vi "Main.vi"() -> ()   [LabVIEW 2015]
uses:
  Share Data/DEVICE_BUSY.ctl
  Share Data/Share Variable.lvlib
panel:
  out "elements":string[](array[string])
  out "Command":string
  out "String 2":string
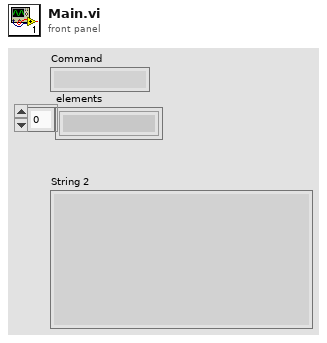
[diagram p1: front panel]
types:
  T1 = typedef "DEVICE_BUSY.ctl" = cluster{"DEV":string, "BUSY":bool, "VBAT":dbl, "OUTPUT":bool, "LAST_RESULT":dbl}
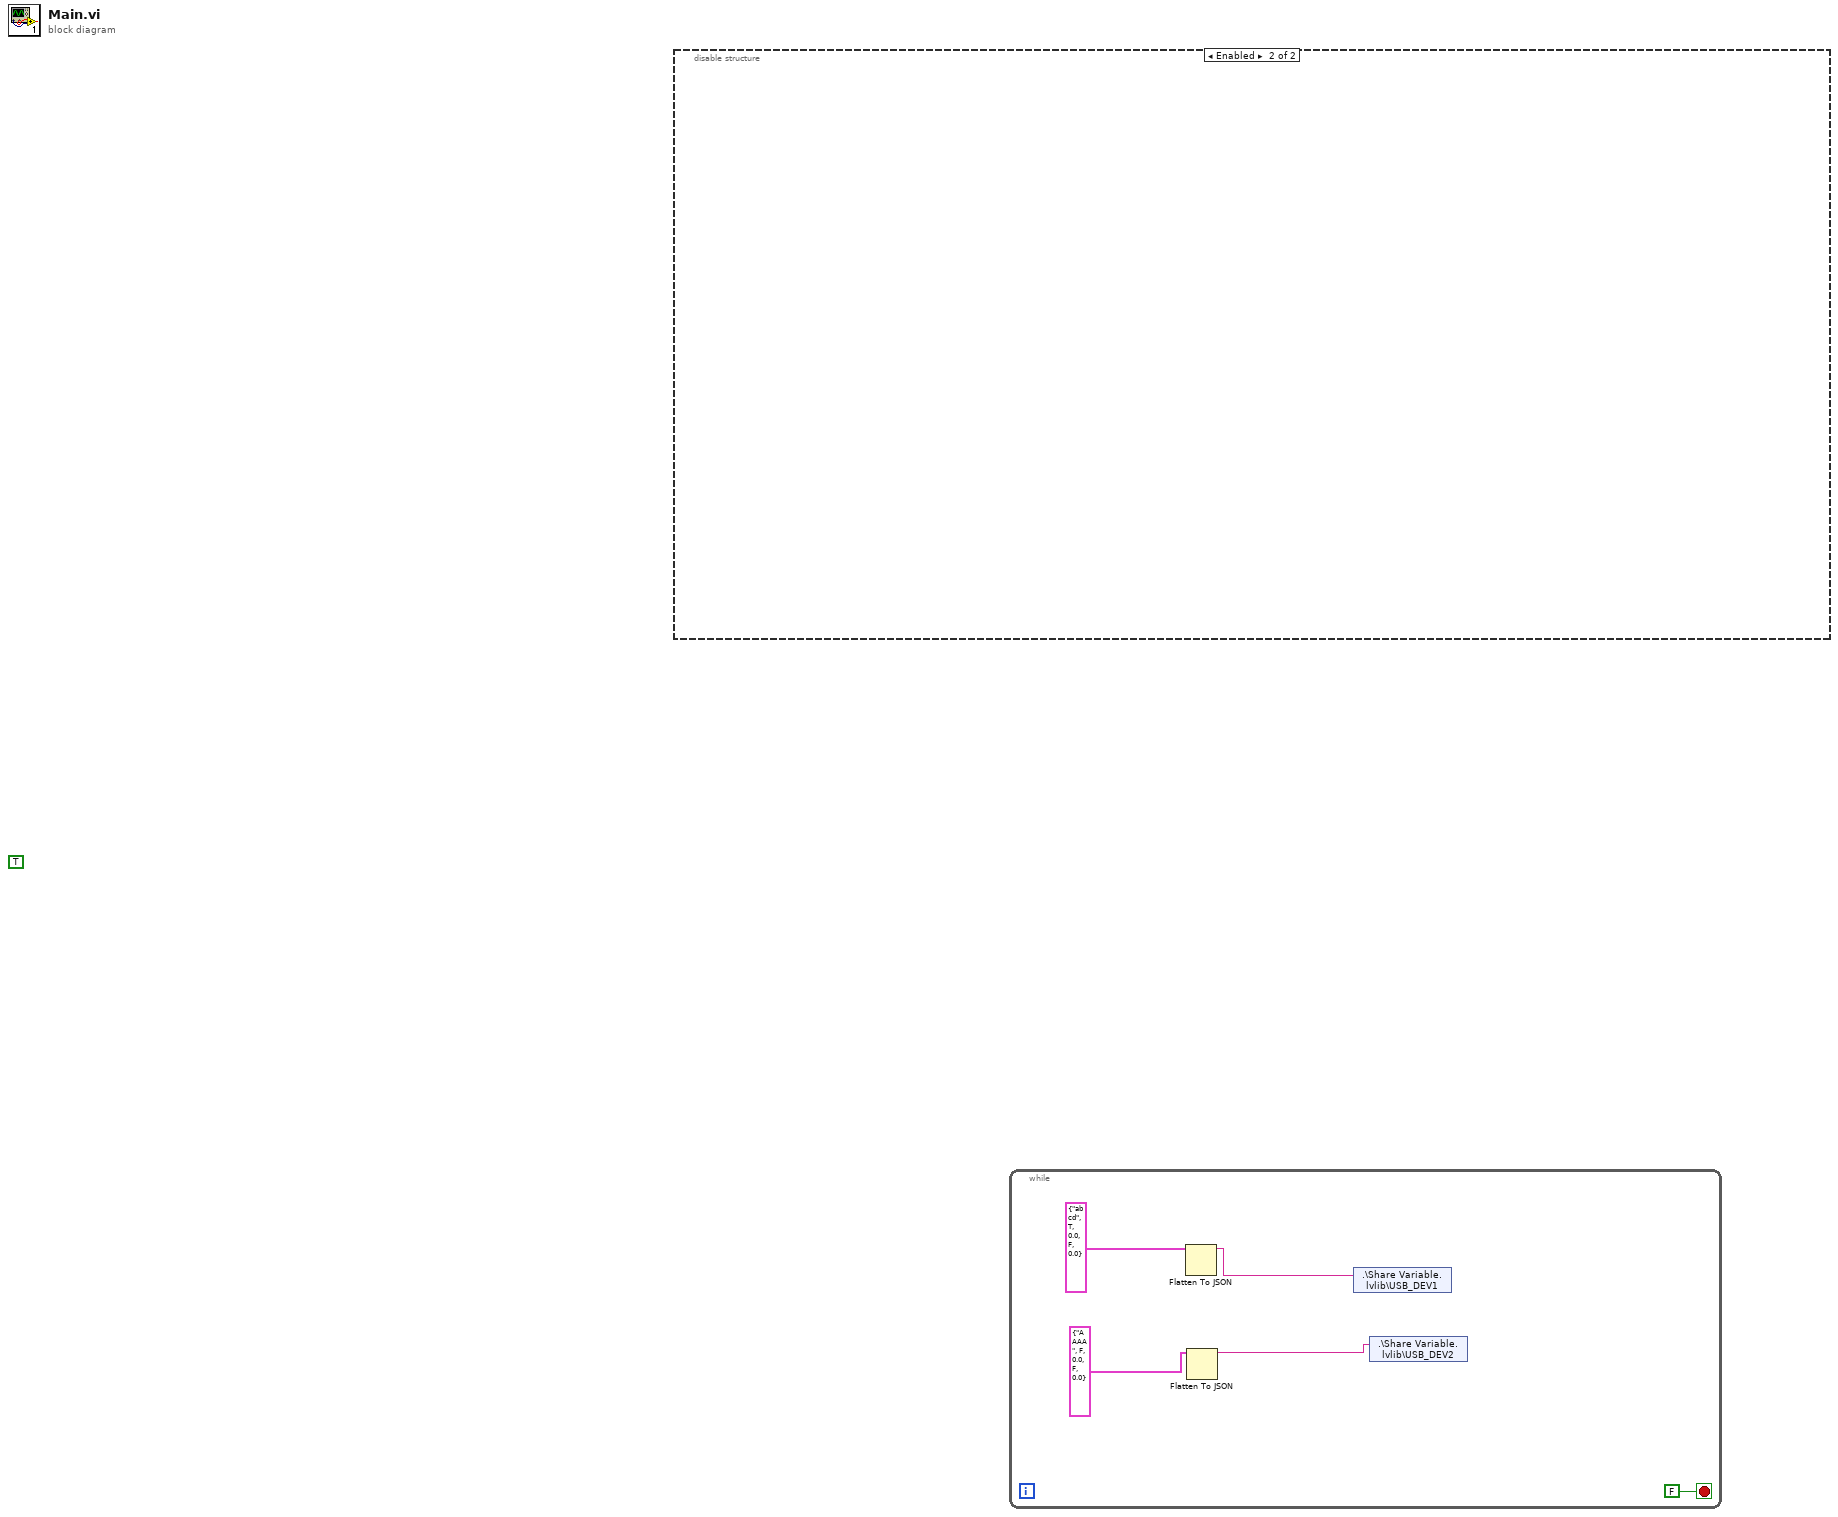
[diagram p0: block diagram]
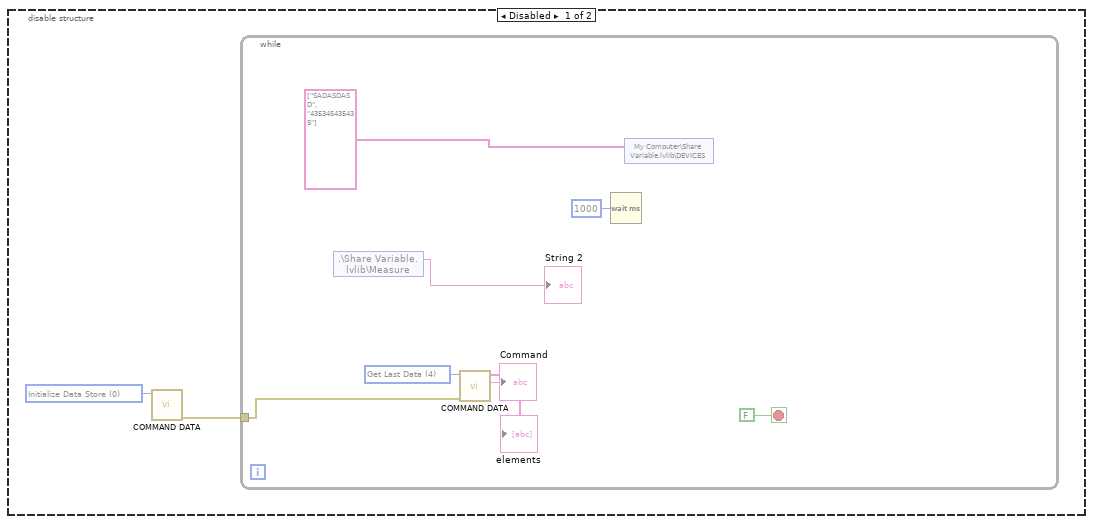
[diagram p2: hidden frame]
diagram:
  (unwired) TRUE
  n1 = disable-structure shown="Enabled" {
    frame Disabled {
      w2 = u16 0 items=["Initialize Data Store", "Destroy Data Store", "Clear Data", "Append Data", "Get Last Data", "Get All Data"] ("action")
      n2 = call "COMMAND DATA.vi"("action"=w2) -> ("error out"=w1:errorcluster)  [unwired: 8 in, 2 out]
      n3 = while {
        tunnel: w1 -> [w6]
        stop <- FALSE stop-if-true
        w5 = u16 4 items=["Initialize Data Store", "Destroy Data Store", "Clear Data", "Append Data", "Get Last Data", "Get All Data", "Waiting - Get  Data"] ("action")
        n4 = shared-variable ".\\Share Variable.lvlib\\Measure"() -> (→"String 2":string)  [unwired: 1 in, 1 out]
        n5 = call "COMMAND DATA.vi"("error in (no error)"=w6, "action"=w5) -> ("Command"=→"Command":string, "elements"=→"elements":string[])  [unwired: 7 in, 1 out]
        n6 = Wait (ms)(milliseconds to wait=u32 1000) -> ()  [unwired: 1 out]
        n7 = shared-variable "My Computer\\Share Variable.lvlib\\DEVICES"(string[] ["SADASDASD", "435345435435"] ("DEVICES")) -> ()  [unwired: 1 in, 1 out]
      }
    }
    frame Enabled {
    }
  }
  n8 = while {
    stop <- FALSE stop-if-true
    n9 = Flatten To JSON(anything=T1 {"DEV"="abcd", "BUSY"=TRUE, "VBAT"=0.0, "OUTPUT"=FALSE, "LAST_RESULT"=0.0} ("DEV_BUSY")) -> (JSON string=w13:string)  [unwired: 2 in, 1 out]
    n10 = Flatten To JSON(anything=T1 {"DEV"="AAAA", "BUSY"=FALSE, "VBAT"=0.0, "OUTPUT"=FALSE, "LAST_RESULT"=0.0} ("DEV_BUSY")) -> (JSON string=w11:string)  [unwired: 2 in, 1 out]
    n11 = shared-variable ".\\Share Variable.lvlib\\USB_DEV1"(w13) -> ()  [unwired: 1 in, 1 out]
    n12 = shared-variable ".\\Share Variable.lvlib\\USB_DEV2"(w11) -> ()  [unwired: 1 in, 1 out]
  }
